vi "Apply Settings.vi"(8 "error in (no error)":errorcluster, 11 "VacuumLines in":refnum<class "VacuumLines.lvclass">) -> (0 "error out":errorcluster, 3 "VacuumLines out":refnum<class "VacuumLines.lvclass">)   [LabVIEW 2016, in "Hardware.lvlib" / "VacuumLine.lvlib" / "VacuumLines.lvclass"]
uses:
  <userlib>/Common Components/Hardware/Abstract System/VacuumLine/VacuumLines/VacuumLines.lvclass
  <userlib>/Common Components/Hardware/Abstract System/VacuumLine/VacuumLines/VacuumLines.lvclass/VacuumLines.ctl
  <userlib>/Common Components/Hardware/Abstract System/VacuumLine/VacuumLine/VacuumLine.lvclass/VacuumLine.ctl
  <userlib>/Common Components/Hardware/LogicIO/LogicIO/Dummy Data.ctl
  <userlib>/Common Components/Hardware/Abstract System/VacuumLine/VacuumLine/Valve Complex.ctl
  <userlib>/Common Components/Hardware/Abstract System/VacuumLine/VacuumLine/Logic Cluster.ctl
  <userlib>/Common Components/Hardware/LogicIO/LogicIO/LogicIO.lvclass
  <userlib>/Common Components/Hardware/Abstract System/VacuumLine/VacuumLine/VacuumLine.lvclass
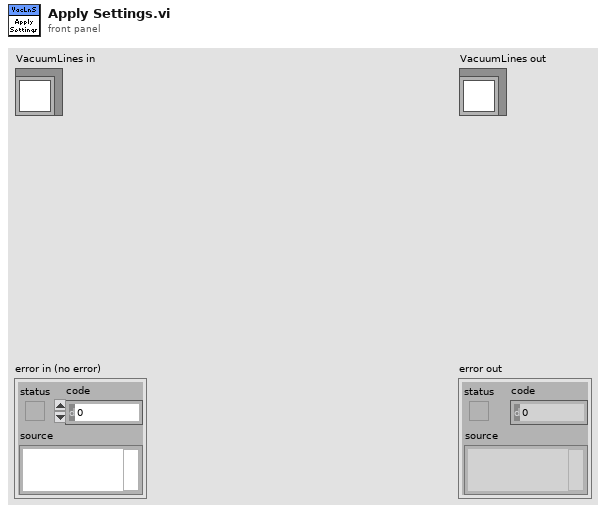
[diagram p1: front panel]
types:
  T1 = typedef "Hardware.lvlib/LogicIO.lvlib/LogicIO.lvclass/Dummy Data.ctl" = cluster{"Valve Complexes":T2[]}
  T2 = typedef "Hardware.lvlib/VacuumLine.lvlib/VacuumLine.lvclass/Valve Complex.ctl" = cluster{"LogicIO Module":string, "Valve Open":T3, "Optical Switch -":T3, "Optical Switch +":T3, "Valve Closed Status Alert":cluster{"Pin#":u8, "Option":enum16{"Not Used", "Normally Closed"}}}
  T3 = typedef "Hardware.lvlib/VacuumLine.lvlib/VacuumLine.lvclass/Logic Cluster.ctl" = cluster{"Pin#":u8, "Location":dbl, "Tolerance":dbl}
  T4 = typedef "Hardware.lvlib/VacuumLine.lvlib/VacuumLine.lvclass/VacuumLine Params.ctl" = cluster{"Motion Limits":cluster{"min":dbl, "max":dbl}, "No. of Conflict Zones":u8, "Conflict Zones (mm)":cluster{"with":string, "from":dbl, "to":dbl, "buffer":dbl}[], "Valve Complexes":T2[], "max( |Motor Pos - LRF Distance| )":dbl}
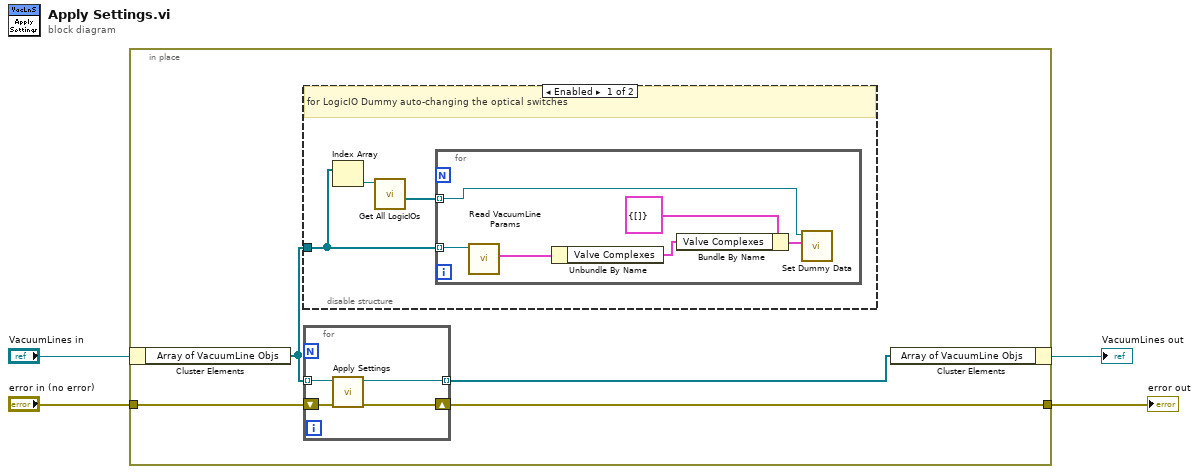
[diagram p0: block diagram]
diagram:
  n1 = in-place {
    in-place-border: "error in (no error)" -> [w7]
    in-place-border: [w6] -> w1
    n2 = in-place-cluster #1("VacuumLines in") -> ("Array of VacuumLine Objs"=w5:refnum<class "VacuumLine.lvclass">[])
    n3 = disable-structure shown="Enabled" {
      disable-tunnel: w5 -> [w9 _]
      frame Enabled {
        # "for LogicIO Dummy auto-changing the optical switches"
        n4 = Index Array(array=w9) -> (element=w11:refnum<class "VacuumLine.lvclass">)  [unwired: 1 in]
        n5 = call <userlib>:"Get All LogicIOs.vi"("VacuumLine in"=w11) -> ("LogicIOs"=w10:refnum<class "LogicIO.lvclass">[])  [unwired: 7 in, 3 out]
        n6 = for {
          tunnel: w10 -> [w15] mode=indexing
          tunnel: w9 -> [w17] mode=indexing
          n7 = call <userlib>:"Read VacuumLine Params.vi"("VacuumLine in"=w17) -> ("Position Params"=w16:T4)  [unwired: 8 in, 2 out]
          n8 = Unbundle By Name(w16) -> ("Valve Complexes"=w12:T2[])
          n9 = Bundle By Name(cluster=T1 {"Valve Complexes"=[]} ("Dummy Data"), "Valve Complexes"=w12) -> (w13:T1)
          n10 = call-dynamic "Set Dummy Data.vi"("Dummy Data"=w13, "LogicIO in"=w15) -> ()  [unwired: 8 in, 2 out]
        }
      }
      frame Disabled {
      }
    }
    n11 = for {
      tunnel: w5 -> [w21] mode=indexing
      tunnel: [w20] -> w8 mode=indexing
      shift-right: [w18] -> w6
      shift-left: w7 -> [w19]
      n12 = call <userlib>:"Apply Settings.vi"("error in (no error)"=w19, "VacuumLine in"=w21) -> ("error out"=w18:errorcluster, "VacuumLine out"=w20:refnum<class "VacuumLine.lvclass">)  [unwired: 8 in]
    }
    n13 = in-place-cluster #1("Array of VacuumLine Objs"=w8) -> (→"VacuumLines out":refnum<class "VacuumLines.lvclass">)
  }
  "error out" <- w1
